vi "Test Z Set-Point Number of Samples Calculation.vi"() -> (0 "Reason":string, 1 "Success":bool)   [LabVIEW 2013]
uses:
  <vilib>/xml/Load XML File.vi
  <vilib>/xml/NI_XML.lvlib
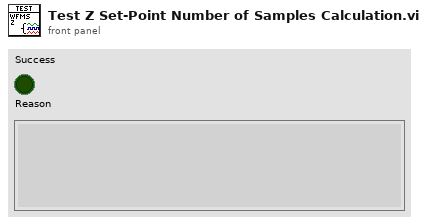
[diagram p1: front panel]
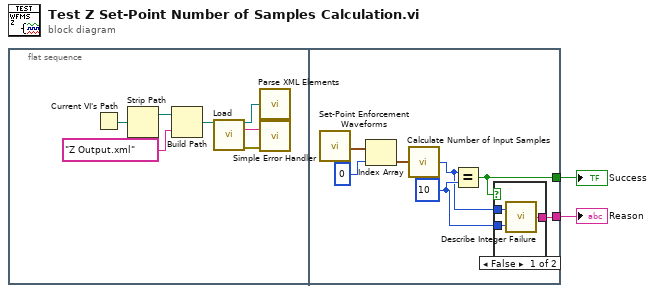
[diagram p0: block diagram]
diagram:
  n1 = flat-sequence {
    tunnel: [w13] -> w2
    tunnel: [w12] -> w1
    frame #0 {
      n2 = Current VI's Path() -> (path=w9:path)
      n3 = Strip Path(path=w9) -> (stripped path=w8:path)  [unwired: 1 out]
      n4 = Build Path(base path=w8, name or relative path="Z Output.xml") -> (appended path=w3:path)
      n5 = call-poly <vilib>:"Load.vi"("path to XML document"=w3) -> ("DOM document out"=w6:refnum<k20>, "parse errors"=w4:string, "error out"=w5:errorcluster)  [unwired: 12 in]
      n6 = call "Parse XML Elements.vi"("DOM"=w6) -> ()
      n7 = call <vilib>:"Simple Error Handler.vi"("error source (\" \")"=w4, "error in (no error)"=w5) -> ()  [unwired: 3 in, 5 out]
    }
    frame #1 {
      w11 = 10 ("y")
      n8 = call "Set-Point Enforcement Waveforms.vi"() -> ("Output Waveforms"=w16:waveform(dbl)[])
      n9 = Index Array(array=w16, index=0) -> (element=w14:waveform(dbl))
      n10 = call "Calculate Number of Input Samples.vi"("Output Waveform"=w14) -> ("Number Of Samples"=w10:i32)
      n11 = Equal?(x=w10, y=w11) -> (x = y?=w13:bool)
      n12 = case shown="False" w13 {
        tunnel: [w19 _] -> w12
        tunnel: w11 -> [w18 _]
        tunnel: w10 -> [w17 _]
        frame False {
          n13 = call "Describe Integer Failure.vi"("Expected"=w18, "Got"=w17) -> ("Failure Description"=w19:string)
        }
        frame True {
        }
      }
    }
  }
  "Success" <- w2
  "Reason" <- w1
